vi "Filter VI Key Down Event.vi"(8 "error in (no error)":errorcluster, 10 "VIKeyDownMsg":refnum<class "VIKeyDownMsg.lvclass">, 11 "IEventFilter in":refnum<class "IEventFilter.lvclass">) -> (0 "error out":errorcluster, 1 "Discard?":bool, 2 "Filtered Event Data":T2, 3 "IEventFilter out":refnum<class "IEventFilter.lvclass">, 5 "Data Filtered?":bool)   [LabVIEW 2020, in "ActorEvents.lvlib" / "IEventFilter.lvclass"]
uses:
  IEventFilter.lvclass
  IEventFilter.lvclass/IEventFilter.ctl
  <vilib>/event_ctls.llb/eventvkey.ctl
  IEventAggregator Messages/VIKeyDownMsg/VIKeyDownMsg.lvclass
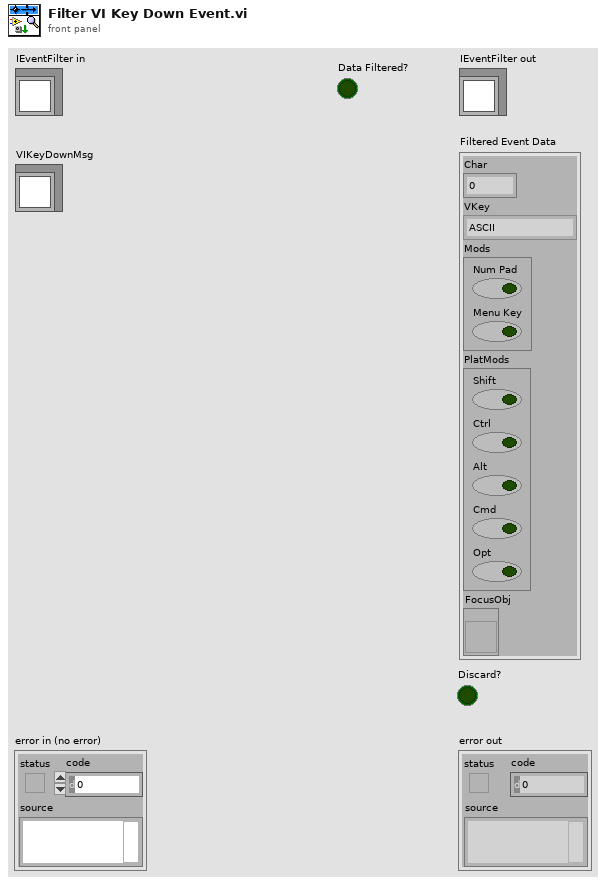
[diagram p1: front panel]
types:
  T1 = typedef "eventvkey.ctl" = enum16{"ASCII", "Enter", "Return", "Shift", "Ctrl", "Alt", "Cmd", "Opt", "Caps", "NumLock", "Clear", "Break", "Up", "Down", "Left", "Right", "Insert", "Delete", "Home", "End", "PageUp", "PageDown", "Escape", "Help", "Pause", "ScrollLock", "F1", "F2", "F3", "F4", "F5", "F6", "F7", "F8", "F9", "F10", "F11", "F12", "F13", "F14", "F15", "F16", "F17", "F18", "F19", "F20", "F21", "F22", "F23", "F24", "Play", "VolumeUp", "VolumeDown", "Mute", "Two Byte Char"}
  T2 = cluster{"Char":i16, "VKey":T1, "Mods":cluster{"Num Pad":bool, "Menu Key":bool}, "PlatMods":cluster{"Shift":bool, "Ctrl":bool, "Alt":bool, "Cmd":bool, "Opt":bool}, "FocusObj":refnum<vi>}
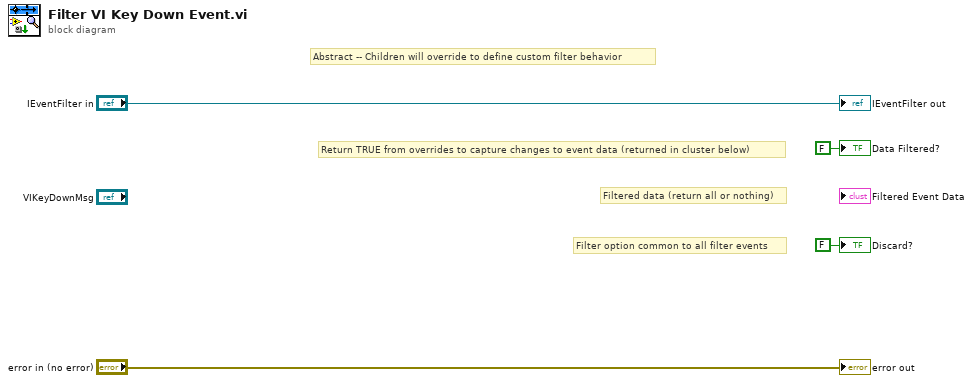
[diagram p0: block diagram]
diagram:
  # "Filtered data (return all or nothing)"
  # "Filter option common to all filter events"
  # "Return TRUE from overrides to capture changes to event data (returned in cluster below)"
  # "Abstract -- Children will override to define custom filter behavior"
  "error out" <- "error in (no error)"
  "IEventFilter out" <- "IEventFilter in"
  "Discard?" <- FALSE ("Discard?")
  "Data Filtered?" <- FALSE ("Data Filtered?")
